vi "Autocorr_sub.vi"(5 "Freeform":T1={"model"="((1/n)*(1+(r/(1-r))*exp(-x/t1))/(1+x/t2)*(1+x/(4*t2))^(-1/2))+o", "Parameters"=["o", "t1", "t2", "n", "r"], "x"="x"}, 6 "skip":i32, 7 "Substitution Rules":T2(array[cluster]), 8 "min bin time (ns)":u32=1000, 9 "MacroTimes":i32[](array[numeric]), 10 "Initial Guess Coefficient":dbl[](array[numeric])=[0.0, 0.001, 1.0, 0.8, 0.5] format="%.2e", 11 "Fit-Type":u8=1) -> (0 "off":dbl format="%.2f", 1 "on":dbl format="%.2f", 2 "Autocorr 2":cluster{dbl[], "Best Fit":dbl[]}[](graph), 3 "Deviation":cluster{dbl[], dbl[]}(graph), 4 "Best Fit Coefficients":dbl[](array[numeric]) format="%.2e")   [LabVIEW 2009]
uses:
  <vilib>/gmath/NI_Gmath.lvlib
panel:
  out "Parameters":string[](array[string])
  out "Parameters":string[](array[string])
  in  "max iteration":i32=200
  out "error":i32
  out "Diffusion":T1={"model"="(1/N) * (1 + ((Teq / (1-Teq)) * exp(-x/tt)))", "Parameters"=["tt", "N", "Teq"], "x"="x"}
  in  "n: fit-channels":i32=800
  out "Autocorr 3":cluster{dbl[], dbl[]}[](graph)=[{[0.001, 0.002, 0.003, 0.004, 0.005, 0.006, 0.006999999999999999, 0.008], [0.3056130111217499, 0.1263820379972458, 0.2014741748571396, 0.19662952423095703, 0.14333832263946533, 0.16029462218284607, 0.23175325989723206, 0.16271694004535675]}, {[0.01, 0.012, 0.013999999999999999, 0.016], [0.1814902424812317, 0.20268559455871582, 0.1814902424812317, 0.19602419435977936]}, {[0.02, 0.024, 0.027999999999999997, 0.032], [0.2011716514825821, 0.1972353607416153, 0.1684892326593399, 0.17727030813694]}, {[0.04, 0.048, 0.055999999999999994, 0.064], [0.16262252628803253, 0.18639276921749115, 0.18654417991638184, 0.16686180233955383]}, {[0.08, 0.096, 0.11199999999999999, 0.128], [0.189042329788208, 0.1808665692806244, 0.15732342004776, 0.17503756284713745]}, {[0.16, 0.192, 0.22399999999999998, 0.256], [0.16345523297786713, 0.17848245799541473, 0.1583830714225769, 0.1600295752286911]}, {[0.32, 0.384, 0.44799999999999995, 0.512], [0.15505988895893097, 0.15379180014133453, 0.15740670263767242, 0.15239104628562927]}, {[0.64, 0.768, 0.8959999999999999, 1.024], [0.14732517302036285, 0.14066201448440552, 0.1391477733850479, 0.14085091650485992]}, {[1.28, 1.536, 1.7919999999999998, 2.048], [0.1371297538280487, 0.137104794383049, 0.1373547464609146, 0.13686597347259521]}, {[2.56, 3.072, 3.5839999999999996, 4.096], [0.13611261546611786, 0.12637928128242493, 0.12281469255685806, 0.11785545945167542]}, {[5.12, 6.144, 7.167999999999999, 8.192], [0.1232251301407814, 0.11928267776966095, 0.12052332609891891, 0.12087620794773102]}, {[10.24, 12.288, 14.335999999999999, 16.384], [0.11623159050941467, 0.11148574203252792, 0.11051606386899948, 0.11171012371778488]}, {[20.48, 24.576, 28.671999999999997, 32.768], [0.09840060025453568, 0.09445063769817352, 0.08400378376245499, 0.08272682130336761]}, {[40.96, 49.152, 57.343999999999994, 65.536], [0.06040594354271889, 0.04272511973977089, 0.03144429251551628, 0.020498599857091904]}, {[81.92, 98.304, 114.68799999999999, 131.072], [0.005955248139798641, -8.516249363310635e-05, -0.004393902141600847, -0.0032490675803273916]}, {[163.84, 196.608, 229.37599999999998, 262.144], [0.00481762457638979, 0.006476061884313822, 0.00663176691159606, 0.008486073464155197]}, {[327.68, 393.216, 458.75199999999995, 524.288], [0.005188951268792152, 0.006893649231642485, 0.008972695097327232, 0.0029570164624601603]}]
  # "1/N * (1+(Teq/(1-Teq)*exp(-x/tt))) * (1+x/tc)^(-1)*(1+x/((K^2)*tc))^(0.5) + o"
  # "y=1.2*(1+0.2/(1-0.2)*exp(-x/5E-7))*(1+x/(2E-4))**(-1)*(1+x/(4**2*(2E-4)))**(-0.5);"
  # "Exponenential"
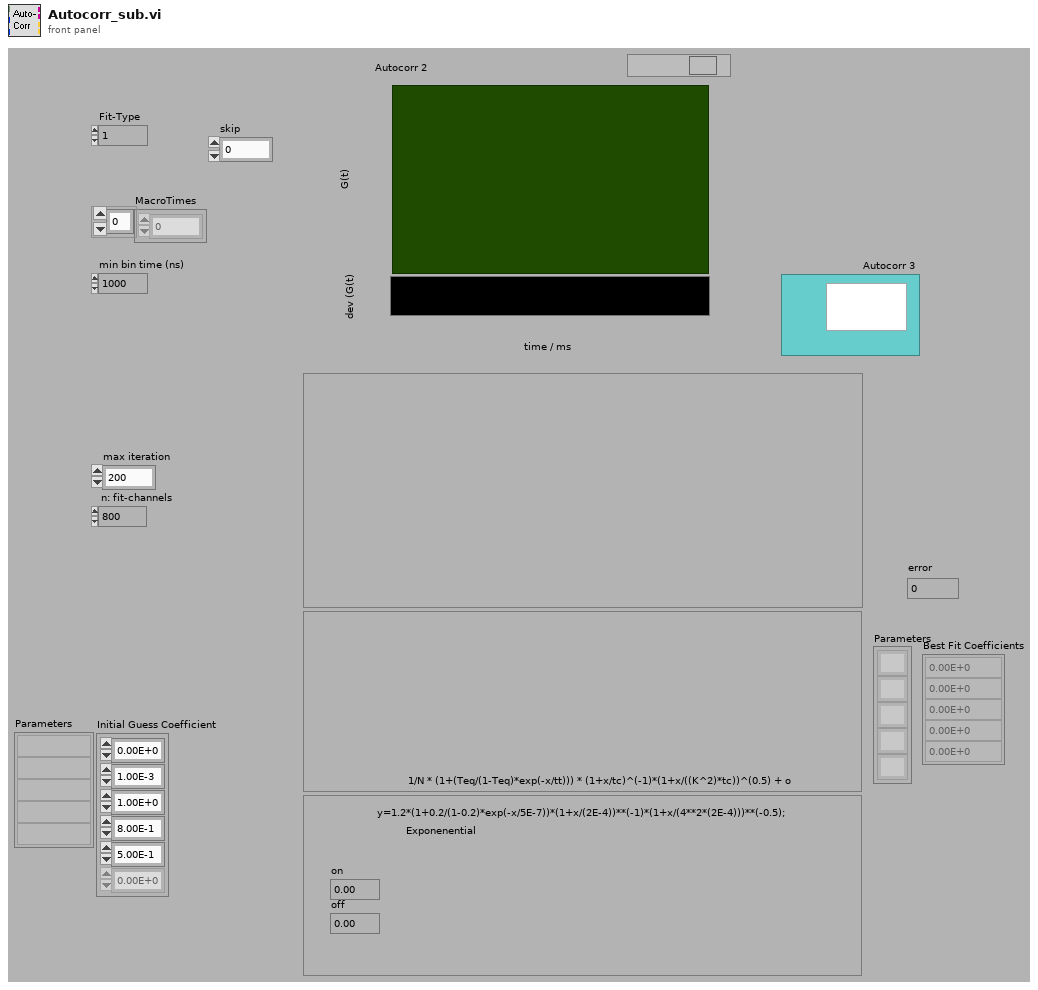
[diagram p1: front panel]
types:
  T1 = cluster{"model":string, "Parameters":string[], "x":string}
  T2 = cluster{"parameter name":string, "parameter content":string}[]
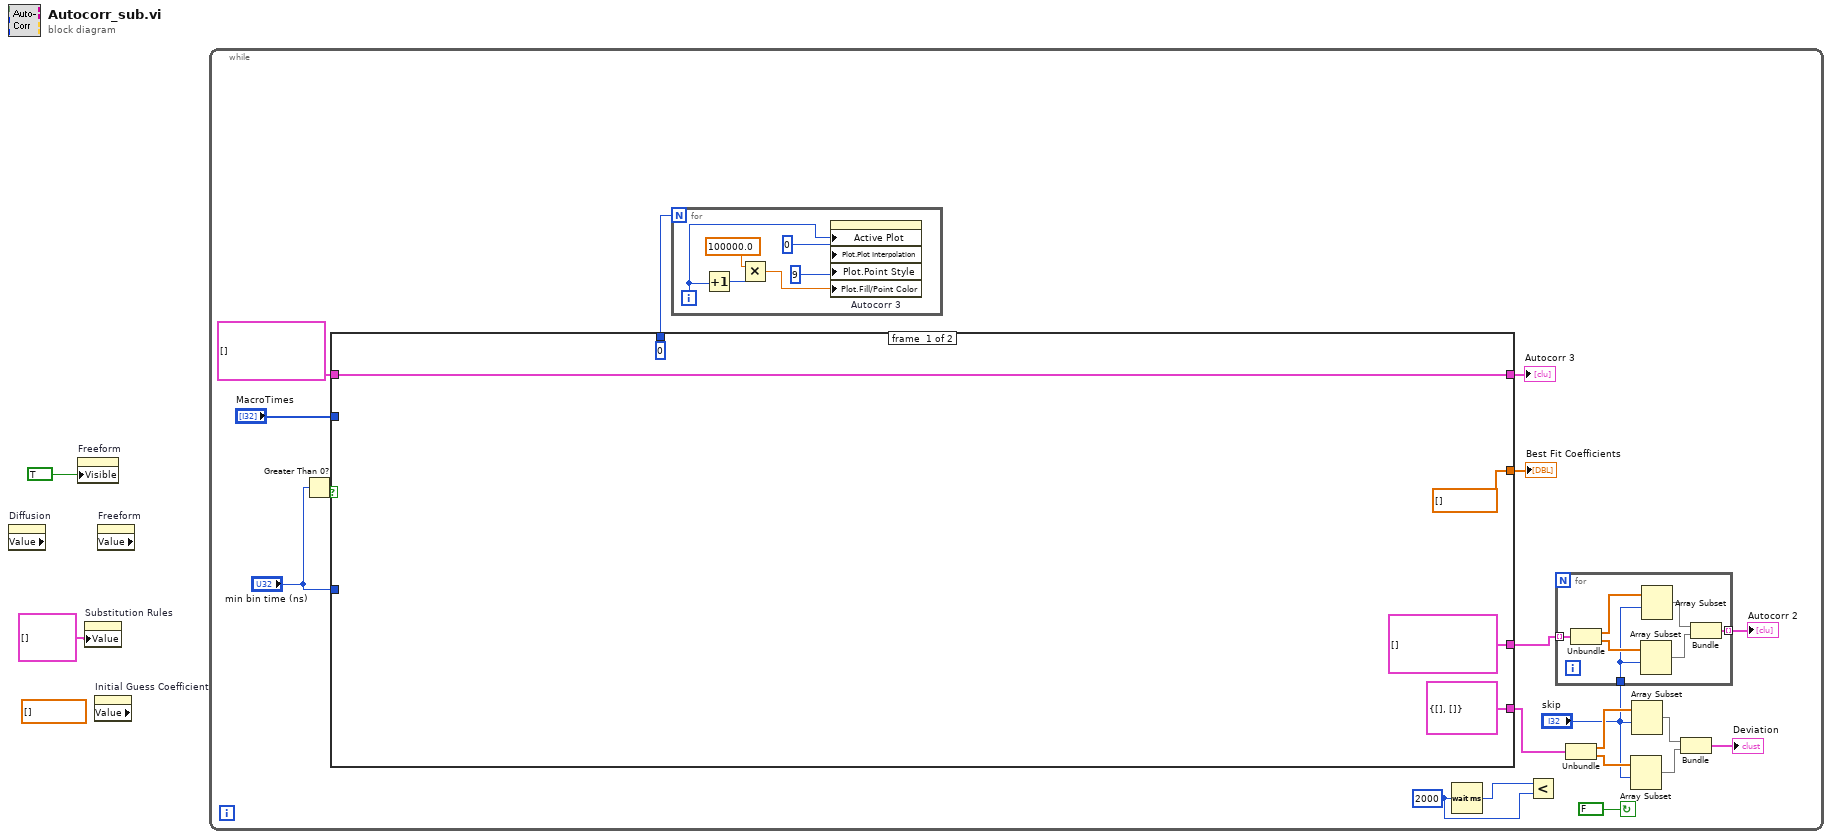
[diagram p0: block diagram]
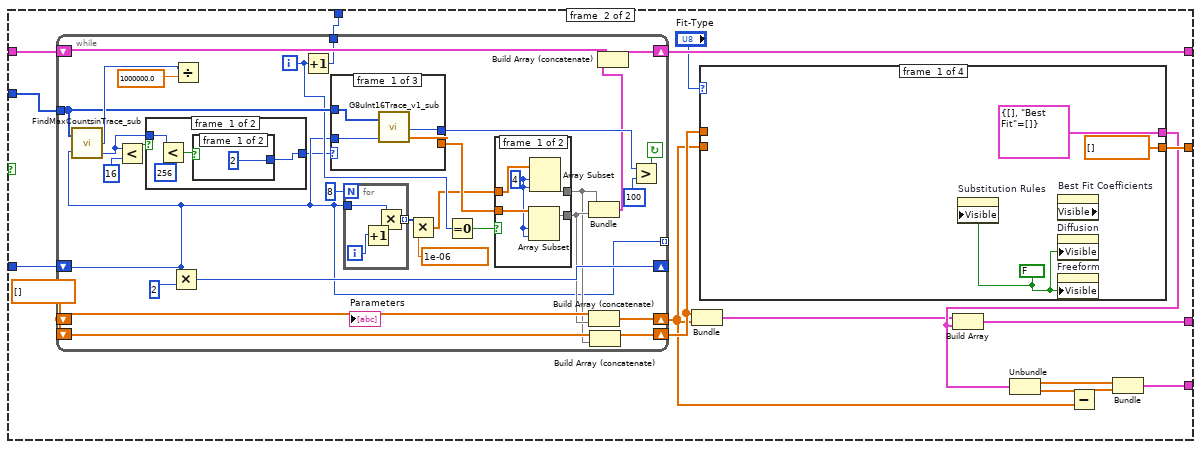
[diagram p2: hidden frame]
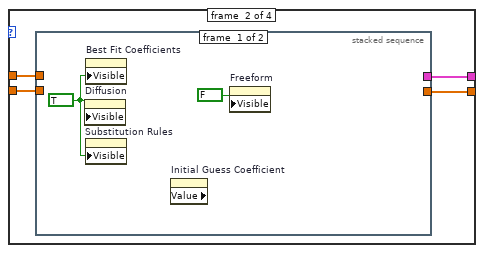
[diagram p3: hidden frame]
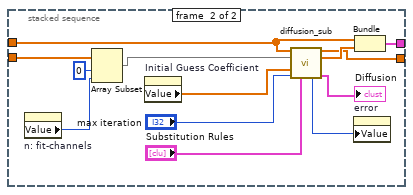
[diagram p4: hidden frame]
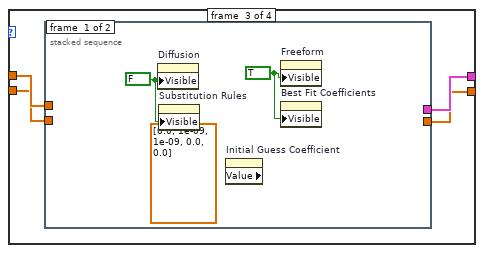
[diagram p5: hidden frame]
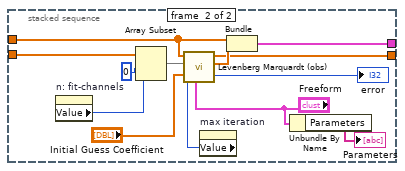
[diagram p6: hidden frame]
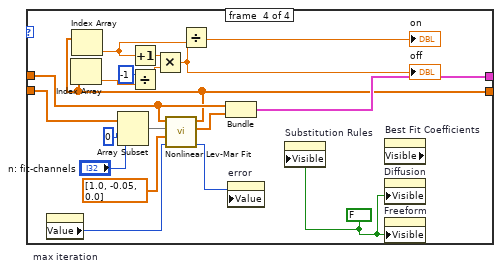
[diagram p7: hidden frame]
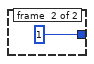
[diagram p9: hidden frame]
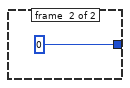
[diagram p10: hidden frame]
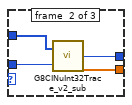
[diagram p11: hidden frame]
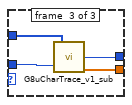
[diagram p12: hidden frame]
diagram:
  (unwired) dbl[] [] ("Initial Guess Coefficient")
  n1 = property on="Diffusion" class="Cluster (strict)" props=["Value"]() -> ()  [unwired: 2 in, 3 out]
  n2 = property on="Freeform" class="Cluster (strict)"("Visible"=TRUE) -> ()  [unwired: 2 in, 2 out]
  n3 = property on="Substitution Rules" class="Array (strict)"("Value"=T2 [] ("Substitution Rules")) -> ()  [unwired: 2 in, 2 out]
  n4 = property on="Initial Guess Coefficient" class="Array (strict)" props=["Value"]() -> ()  [unwired: 2 in, 3 out]
  n5 = property on="Freeform" class="Cluster (strict)" props=["Value"]() -> ()  [unwired: 2 in, 3 out]
  n6 = while {
    stop <- FALSE continue-if-true
    w12 = u32 2000 ("milliseconds to wait")
    n7 = Greater Than 0?(x="min bin time (ns)") -> (x > 0?=w18:bool)
    n8 = case shown="True" w18 {
      tunnel: "min bin time (ns)" -> [_ w56]
      tunnel: cluster{dbl[], dbl[]}[] [] -> [w38 w55]
      tunnel: [0 w54] -> w20
      tunnel: "MacroTimes" -> [_ w52]
      tunnel: [w38 w51] -> w16
      tunnel: [cluster{dbl[], "Best Fit":dbl[]}[] [] w50] -> w11
      tunnel: [dbl[] [] ("Best Fit Coefficients") w48] -> w15
      tunnel: [cluster{dbl[], dbl[]} {[], []} w42] -> w5
      frame #0 {
      }
      frame #1 {
        w53 = dbl[] []
        n9 = while {
          tunnel: [w123] -> _ mode=indexing
          tunnel: w52 -> [w128]
          shift-left: w53 -> [w129]
          shift-right: [w130] -> w47
          shift-left: w53 -> [w131]
          shift-right: [w132] -> w45
          tunnel: [w137] -> w54
          shift-left: w56 -> [w123]
          shift-right: [w144] -> _
          shift-left: w55 -> [w143]
          shift-right: [w146] -> w51
          i -> [w127]
          stop <- w138 continue-if-true
          n10 = call "FindMaxCountsinTrace_sub.vi"("Macros"=w128, "bin time (ns)"=w123) -> ("tracelength"=w133:i32, "max counts"=w121:i32)  [unwired: 1 out]
          n11 = Less?(x=w121, y=16) -> (x < y?=w135:bool)
          n12 = case shown="False" w135 {
            tunnel: [w154 0] -> w122
            tunnel: w121 -> [w157 _]
            frame #0 {
              n13 = Less?(x=w157, y=256) -> (x < y?=w155:bool)
              n14 = case shown="True" w155 {
                tunnel: [2 1] -> w154
                frame #0 {
                }
                frame #1 {
                }
              }
            }
            frame #1 {
            }
          }
          n15 = Multiply(x=w123, y=2) -> (x*y=w144:u32)
          n16 = Divide(x=w133, y=1000000.0) -> ()  [unwired: 1 out]
          n17 = Increment(x=w127) -> (x+1=w137:i32)
          n18 = case shown="1" w122 {
            tunnel: [w162 w168 w171] -> w119
            tunnel: w123 -> [w164 w167 w172]
            tunnel: [w163 w165 w170] -> w120
            tunnel: w128 -> [w161 w166 w169]
            frame #0 {
              n19 = call "G8uInt16Trace_v1_sub.vi"("Macros"=w161, "bin time (ns)"=w164) -> ("Trace Length"=w163:i32, "Output Array"=w162:sgl[])  [unwired: 1 out]
            }
            frame #1 {
              n20 = call "G8CINuInt32Trace_v2_sub.vi"("Macros"=w166, "bin time (ns)"=w167) -> ("Trace Length"=w165:i32, "G1-G8"=w168:sgl[])  [unwired: 1 out]
            }
            frame #2 {
              n21 = call "G8uCharTrace_v1_sub.vi"("Macros"=w169, "bin time (ns)"=w172) -> ("Trace Length"=w170:i32, "G1-G8"=w171:sgl[])  [unwired: 1 out]
            }
          }
          n22 = for {
            N: 8 -> [_]
            tunnel: w123 -> [w175]
            tunnel: [w173] -> w141 mode=indexing
            i -> [w176]
            n23 = Increment(x=w176) -> (x+1=w174:i32)
            n24 = Multiply(x=w175, y=w174) -> (x*y=w173:u32)
          }
          n25 = Multiply(x=w141, y=1e-06) -> (x*y=w118:dbl[])
          n26 = Equal To 0?(x=w127) -> (x = 0?=w124:bool)
          n27 = case shown="False" w124 {
            tunnel: w119 -> [w150 w153]
            tunnel: [w147 w153] -> w126
            tunnel: w118 -> [w151 w152]
            tunnel: [w148 w152] -> w125
            frame #0 {
              w149 = 4 ("Array Index")
              n28 = Array Subset(array=w150, index=w149, length=w149) -> (w147:sgl[])
              n29 = Array Subset(array=w151, index=w149, length=w149) -> (w148:dbl[])
            }
            frame #1 {
            }
          }
          n30 = Bundle(w125, "G1-G8"=w126) -> (w117:cluster{dbl[], "G1-G8":sgl[]})  [unwired: 1 in]
          n31 = Build Array (concatenate)(w131, w126) -> (w132:dbl[])
          n32 = Build Array (concatenate)(w129, w125) -> (w130:dbl[])
          n33 = Build Array (concatenate)(w143, w117) -> (w146:cluster{dbl[], "G1-G8":dbl[]}[])
          n34 = Greater?(x=w120, y=100) -> (0:w138:bool)
        }
        n35 = Bundle(w47, w45) -> (w40:cluster{dbl[], dbl[]})  [unwired: 1 in]
        n36 = case shown="0" "Fit-Type" {
          tunnel: w47 -> [_ w63 w81 w105]
          tunnel: w45 -> [_ w62 w80 w104]
          tunnel: [cluster{dbl[], "Best Fit":dbl[]} {[], "Best Fit"=[]} w61 w82 w111] -> w41
          tunnel: [dbl[] [] ("Best Fit Coefficients") w60 w79 w99] -> w48
          frame #0 {
            w59 = FALSE ("Visible")
            n37 = property on="Substitution Rules" class="Array (strict)"("Visible"=w59) -> ()  [unwired: 2 in, 2 out]
            n38 = property on="Best Fit Coefficients" class="Array (strict)" props=["Visible"]() -> ()  [unwired: 2 in, 3 out]
            n39 = property on="Diffusion" class="Cluster (strict)"("Visible"=w59) -> ()  [unwired: 2 in, 2 out]
            n40 = property on="Freeform" class="Cluster (strict)"("Visible"=w59) -> ()  [unwired: 2 in, 2 out]
          }
          frame #1 {
            n41 = stacked-sequence {
              tunnel: w63 -> [_ w75]
              tunnel: w62 -> [_ w70]
              tunnel: [_ w74] -> w61
              tunnel: [_ w73] -> w60
              frame #0 {
                w65 = TRUE ("Visible")
                n42 = property on="Diffusion" class="Cluster (strict)"("Visible"=w65) -> ()  [unwired: 2 in, 2 out]
                n43 = property on="Best Fit Coefficients" class="Array (strict)"("Visible"=w65) -> ()  [unwired: 2 in, 2 out]
                n44 = property on="Substitution Rules" class="Array (strict)"("Visible"=w65) -> ()  [unwired: 2 in, 2 out]
                n45 = property on="Initial Guess Coefficient" class="Array (strict)" props=["Value"]() -> ()  [unwired: 2 in, 3 out]
                n46 = property on="Freeform" class="Cluster (strict)"("Visible"=FALSE) -> ()  [unwired: 2 in, 2 out]
              }
              frame #1 {
                n47 = property on="n: fit-channels" class="Digital (strict)"() -> ("Value"=w72:i32)  [unwired: 2 in, 2 out]
                n48 = Array Subset(array=w70, index=0, length=w72) -> (w69:dbl[])
                n49 = property on="Initial Guess Coefficient" class="Array (strict)"() -> ("Value"=w66:dbl[])  [unwired: 2 in, 2 out]
                n50 = call "diffusion_sub.vi"("X"=w75, "Y"=w69, "Initial Guess Coefficients"=w66, "max iteration"="max iteration", "Substitution Rules"="Substitution Rules") -> ("Best Fit Coefficients"=w73:dbl[], "Best Fit"=w77:dbl[], "error"=w78:i32, "model description"=→"Diffusion":T1)  [unwired: 4 in, 3 out]
                n51 = property on="error" class="Digital (strict)"("Value"=w78) -> ()  [unwired: 2 in, 2 out]
                n52 = Bundle(w75, "Best Fit"=w77) -> (w74:cluster{dbl[], "Best Fit":dbl[]})  [unwired: 1 in]
              }
            }
          }
          frame #2 {
            n53 = stacked-sequence {
              tunnel: [_ w94] -> w82
              tunnel: w81 -> [_ w93]
              tunnel: w80 -> [_ w92]
              tunnel: [_ w90] -> w79
              frame #0 {
                (unwired) dbl[] [0.0, 1e-09, 1e-09, 0.0, 0.0] ("Initial Guess Coefficient")
                w83 = FALSE ("Visible")
                w84 = TRUE ("Visible")
                n54 = property on="Diffusion" class="Cluster (strict)"("Visible"=w83) -> ()  [unwired: 2 in, 2 out]
                n55 = property on="Substitution Rules" class="Array (strict)"("Visible"=w83) -> ()  [unwired: 2 in, 2 out]
                n56 = property on="Initial Guess Coefficient" class="Array (strict)" props=["Value"]() -> ()  [unwired: 2 in, 3 out]
                n57 = property on="Freeform" class="Cluster (strict)"("Visible"=w84) -> ()  [unwired: 2 in, 2 out]
                n58 = property on="Best Fit Coefficients" class="Array (strict)"("Visible"=w84) -> ()  [unwired: 2 in, 2 out]
              }
              frame #1 {
                n59 = property on="n: fit-channels" class="Digital (strict)"() -> ("Value"=w91:i32)  [unwired: 2 in, 2 out]
                n60 = Array Subset(array=w92, index=0 ("Array Index"), length=w91) -> (w97:dbl[])
                n61 = property on="max iteration" class="Digital (strict)"() -> ("Value"=w88:i32)  [unwired: 2 in, 2 out]
                n62 = call <vilib>:"Levenberg Marquardt (obs).vi"("model description"="Freeform", "max iteration"=w88, "Initial Guess Coefficient"="Initial Guess Coefficient", "Y"=w97, "X"=w93) -> ("Best Fit"=w95:dbl[], "Best Fit Coefficients"=w90:dbl[], "error"=→"error":i32)  [unwired: 1 in, 3 out]
                n63 = Bundle(w93, "Best Fit"=w95) -> (w94:cluster{dbl[], "Best Fit":dbl[]})  [unwired: 1 in]
                n64 = Unbundle By Name("Freeform") -> ("Parameters"=→"Parameters":string[])
              }
            }
          }
          frame #3 {
            w101 = FALSE ("Visible")
            n65 = property on="max iteration" class="Digital (strict)"() -> ("Value"=w98:i32)  [unwired: 2 in, 2 out]
            n66 = Array Subset(array=w104, index=0 ("Array Index"), length="n: fit-channels") -> (w106:dbl[])
            n67 = call "Nonlinear Lev-Mar Fit.vi"("max iteration"=w98, "Initial Guess Coefficients"=dbl[] [1.0, -0.05, 0.0], "Y"=w106, "X"=w105) -> ("error"=w100:i32, "Best Fit"=w109:dbl[], "Best Fit Coefficients"=w99:dbl[])  [unwired: 2 in, 2 out]
            n68 = Index Array(array=w99) -> (element=w115:dbl)  [unwired: 1 in]
            n69 = Index Array(array=w99) -> (element=w116:dbl)  [unwired: 1 in]
            n70 = Increment(x=w116) -> (x+1=w113:dbl)
            n71 = Divide(x=-1 ("Array Index"), y=w115) -> (x/y=w112:dbl)
            n72 = Multiply(x=w113, y=w112) -> (x*y=w103:dbl)
            "off" <- w103
            n73 = Divide(x=w103, y=w116) -> (x/y=→"on":dbl)
            n74 = Bundle(w105, "Best Fit"=w109) -> (w111:cluster{dbl[], "Best Fit":dbl[]})  [unwired: 1 in]
            n75 = property on="error" class="Digital (strict)"("Value"=w100) -> ()  [unwired: 2 in, 2 out]
            n76 = property on="Substitution Rules" class="Array (strict)"("Visible"=w101) -> ()  [unwired: 2 in, 2 out]
            n77 = property on="Best Fit Coefficients" class="Array (strict)" props=["Visible"]() -> ()  [unwired: 2 in, 3 out]
            n78 = property on="Diffusion" class="Cluster (strict)"("Visible"=w101) -> ()  [unwired: 2 in, 2 out]
            n79 = property on="Freeform" class="Cluster (strict)"("Visible"=w101) -> ()  [unwired: 2 in, 2 out]
          }
        }
        n80 = Build Array(w40, w41) -> (w50:cluster{dbl[], "Best Fit":dbl[]}[])
        n81 = Unbundle(w41) -> (w43:dbl[], "Best Fit"=w46:dbl[])
        n82 = Subtract(x=w46, y=w45) -> (x-y=w44:dbl[])
        n83 = Bundle(w43, w44) -> (w42:cluster{dbl[], dbl[]})  [unwired: 1 in]
      }
    }
    "Autocorr 3" <- w16
    "Best Fit Coefficients" <- w15
    n84 = for {
      N: w20 -> [_]
      i -> [w30]
      n85 = Increment(x=w30) -> (x+1=w29:i32)
      n86 = Multiply(x=100000.0, y=w29) -> (x*y=w31:dbl)
      n87 = property on="Autocorr 3" class="XYGraph (strict)"("Active Plot"=w30, "Plot.Plot Interpolation"=u8 0 ("Write Attribute"), "Plot.Point Style"=u8 9 ("Write Attribute"), "Plot.Fill/Point Color"=w31) -> ()  [unwired: 2 in, 2 out]
    }
    n88 = Wait (ms)(milliseconds to wait=w12) -> (millisecond timer value=w13:u32)
    n89 = Less?(x=w13, y=w12) -> ()  [unwired: 1 out]
    n90 = for {
      tunnel: w11 -> [w28] mode=indexing
      tunnel: [w23] -> w10 mode=indexing
      tunnel: "skip" -> [w22]
      n91 = Unbundle(w28) -> (w27:dbl[], "Best Fit"=w26:dbl[])
      n92 = Array Subset(array=w26, index=w22) -> (w24:dbl[])  [unwired: 1 in]
      n93 = Array Subset(array=w27, index=w22) -> (w25:dbl[])  [unwired: 1 in]
      n94 = Bundle(w25, w24) -> (w23:cluster{dbl[], dbl[]})  [unwired: 1 in]
    }
    "Autocorr 2" <- w10
    n95 = Unbundle(w5) -> (w9:dbl[], w8:dbl[])
    n96 = Array Subset(array=w8, index="skip") -> (w6:dbl[])  [unwired: 1 in]
    n97 = Array Subset(array=w9, index="skip") -> (w7:dbl[])  [unwired: 1 in]
    n98 = Bundle(w7, w6) -> (→"Deviation":cluster{dbl[], dbl[]})  [unwired: 1 in]
  }
